vi "SV TDMS Get Function Properties.vi"() -> ()   [LabVIEW 2017]
uses:
  <vilib>/addons/_NISVFA/_Shared subVIs/Controls/NI Channel Properties.ctl
panel:
  in  "file path":path
  out "Array":string[][](array[string])
  out "tdms file":refnum<k34>
  in  "error in (no error)":errorcluster
  out "error out":errorcluster
  out "tdms file out":refnum<k34>
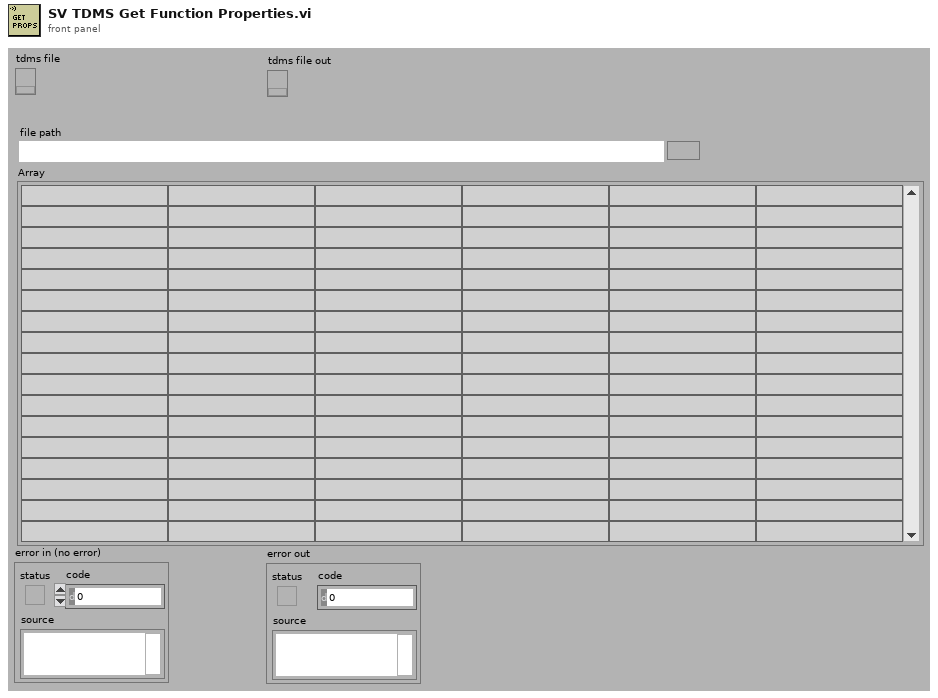
[diagram p1: front panel]
types:
  T1 = typedef "NI Channel Properties.ctl" = u16
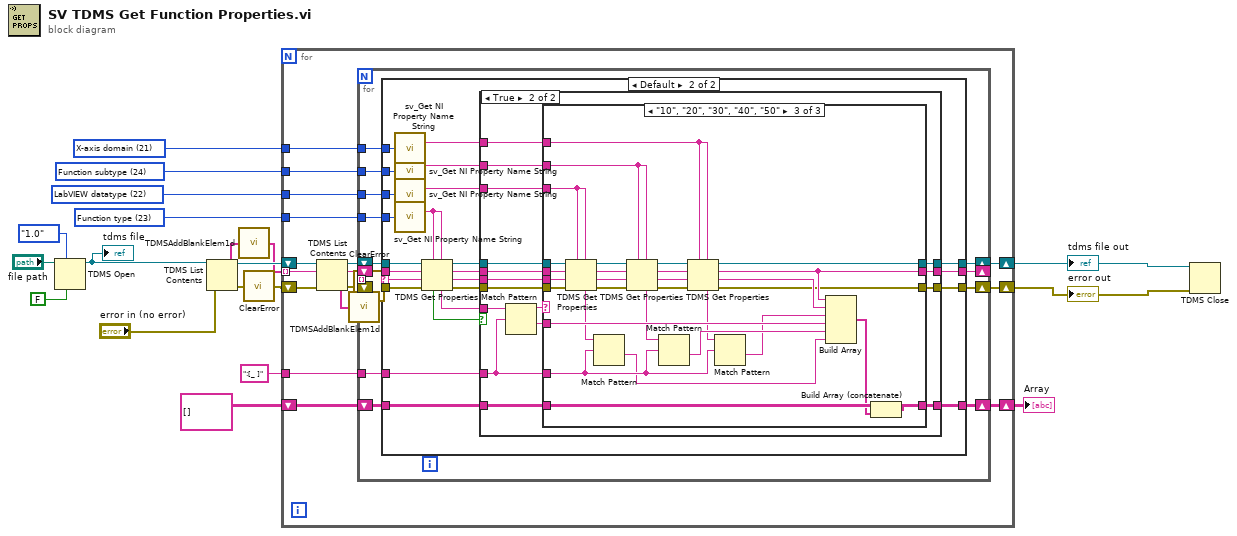
[diagram p0: block diagram]
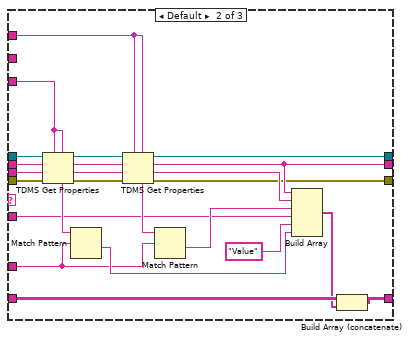
[diagram p5: hidden frame]
diagram:
  w5 = T1 24 items=["Channel name", "Channel description", "Y-axis label", "Y-axis unit string", "X-axis label", "X-axis unit string", "x0", "dx", "Number of samples", "X channel", "Filter settled", "dB reference", "Window", "Window parameter", "Window size", "FFT size", "Peak units", "Spectrum type", "Magnitude scale", "Spectral density", "Sensor sensitivity (mV/EU)", "X-axis domain", "LabVIEW datatype", "Function type", "Function subtype"] ("property")
  w6 = T1 21 items=["Channel name", "Channel description", "Y-axis label", "Y-axis unit string", "X-axis label", "X-axis unit string", "x0", "dx", "Number of samples", "X channel", "Filter settled", "dB reference", "Window", "Window parameter", "Window size", "FFT size", "Peak units", "Spectrum type", "Magnitude scale", "Spectral density", "Sensor sensitivity (mV/EU)", "X-axis domain", "LabVIEW datatype", "Function type", "Component", "Level detector"] ("NI property")
  w7 = T1 22 items=["Channel name", "Channel description", "Y-axis label", "Y-axis unit string", "X-axis label", "X-axis unit string", "x0", "dx", "Number of samples", "X channel", "Filter settled", "dB reference", "Window", "Window parameter", "Window size", "FFT size", "Peak units", "Spectrum type", "Magnitude scale", "Spectral density", "Sensor sensitivity (mV/EU)", "X-axis domain", "LabVIEW datatype", "Function type", "Component", "Level detector"] ("NI property")
  w9 = T1 23 items=["Channel name", "Channel description", "Y-axis label", "Y-axis unit string", "X-axis label", "X-axis unit string", "x0", "dx", "Number of samples", "X channel", "Filter settled", "dB reference", "Window", "Window parameter", "Window size", "FFT size", "Peak units", "Spectrum type", "Magnitude scale", "Spectral density", "Sensor sensitivity (mV/EU)", "X-axis domain", "LabVIEW datatype", "Function type", "Component", "Level detector"] ("NI property")
  n1 = TDMS Open(6:FALSE ("disable buffering? (T)"), 7:enum16{"1.0", "2.0"}."1.0" ("file format version (2.0)"), 11:"file path") -> (3:w10:refnum<k34>)  [unwired: 4 in, 1 out]
  "tdms file" <- w10
  n2 = TDMS List Contents(4:"error in (no error)", 7:w10) -> (0:w1:errorcluster, 2:w2:string[], 3:w19:refnum<k34>)  [unwired: 1 in, 1 out]
  n3 = call <vilib>:"TDMSAddBlankElem1d.vi"("input string array"=w2) -> ("output string array with blank element at the beginning"=w18:string[])
  n4 = call <vilib>:"ClearError.vi"("error in (no error)"=w1) -> ("error out"=w17:errorcluster)
  n5 = for {
    tunnel: w18 -> [w36] mode=indexing
    shift-right: [w33] -> w13
    shift-left: w19 -> [w37]
    shift-right: [w29] -> w14
    shift-left: string[][] [] -> [w30]
    shift-right: [w27] -> w12
    shift-left: w17 -> [w35]
    tunnel: w9 -> [w26]
    tunnel: ":[_ ]" -> [w25]
    tunnel: w7 -> [w24]
    tunnel: w6 -> [w23]
    tunnel: w5 -> [w22]
    n6 = TDMS List Contents(4:w35, 6:w36, 7:w37) -> (0:w20:errorcluster, 1:w21:string[], 2:w31:string, 3:w34:refnum<k34>)
    n7 = call <vilib>:"TDMSAddBlankElem1d.vi"("input string array"=w21) -> ("output string array with blank element at the beginning"=w32:string[])
    n8 = call <vilib>:"ClearError.vi"("error in (no error)"=w20) -> ("error out"=w28:errorcluster)
    n9 = for {
      tunnel: w32 -> [w43] mode=indexing
      shift-right: [w50] -> w33
      shift-left: w34 -> [w51]
      shift-right: [w48] -> _
      shift-left: w31 -> [w49]
      shift-right: [w46] -> w29
      shift-left: w30 -> [w47]
      shift-right: [w44] -> w27
      shift-left: w28 -> [w45]
      tunnel: w26 -> [w42]
      tunnel: w25 -> [w41]
      tunnel: w24 -> [w40]
      tunnel: w23 -> [w39]
      tunnel: w22 -> [w38]
      n10 = case shown="Default" w43 {
        selector: w43 -> [_ w74]
        tunnel: w51 -> [w54 w79]
        tunnel: [w54 w67] -> w50
        tunnel: w49 -> [w55 w78]
        tunnel: [w55 w69] -> w48
        tunnel: w47 -> [w53 w77]
        tunnel: [w53 w76] -> w46
        tunnel: w45 -> [w52 w75]
        tunnel: [w52 w68] -> w44
        tunnel: w42 -> [_ w62]
        tunnel: w41 -> [_ w63]
        tunnel: w40 -> [_ w61]
        tunnel: w39 -> [_ w59]
        tunnel: w38 -> [_ w57]
        frame "" {
        }
        frame Default {
          n11 = call <vilib>:"sv_Get NI Property Name String.vi"("property"=w59) -> ("TDMS property name"=w58:string)  [unwired: 13 in, 1 out]
          n12 = call <vilib>:"sv_Get NI Property Name String.vi"("property"=w57) -> ("TDMS property name"=w56:string)  [unwired: 13 in, 1 out]
          n13 = call <vilib>:"sv_Get NI Property Name String.vi"("property"=w61) -> ("TDMS property name"=w60:string)  [unwired: 13 in, 1 out]
          n14 = call <vilib>:"sv_Get NI Property Name String.vi"("property"=w62) -> ("TDMS property name"=w66:string)  [unwired: 13 in, 1 out]
          n15 = TDMS Get Properties(5:w66, 7:w66, 8:w75, 9:w74, 10:w78, 11:w79) -> (0:w73:errorcluster, 1:w72:string, 2:w71:string, 3:w70:refnum<k34>, 4:w64:string, 6:w65:bool)
          n16 = case shown="True" w65 {
            tunnel: w77 -> [w83 w99]
            tunnel: [w83 w98] -> w76
            tunnel: w73 -> [w82 w97]
            tunnel: w72 -> [_ w96]
            tunnel: w71 -> [w81 w95]
            tunnel: w70 -> [w80 w94]
            tunnel: [w81 w93] -> w69
            tunnel: [w82 w92] -> w68
            tunnel: [w80 w91] -> w67
            tunnel: w64 -> [_ w87]
            tunnel: w63 -> [_ w86]
            tunnel: w60 -> [_ w89]
            tunnel: w58 -> [_ w88]
            tunnel: w56 -> [_ w84]
            frame False {
            }
            frame True {
              n17 = Match Pattern(string=w87, regular expression=w86) -> (before substring=w90:string, after substring=w85:string)  [unwired: 1 in, 2 out]
              n18 = case shown="\"10\", \"20\", \"30\", \"40\", \"50\"" w90 {
                tunnel: w99 -> [w100 w127 w157]
                tunnel: [w100 w126 w156] -> w98
                tunnel: w97 -> [w101 w117 w155]
                tunnel: w96 -> [_ w118 w154]
                tunnel: w95 -> [w102 w119 w153]
                tunnel: w94 -> [w103 w120 w152]
                tunnel: [w102 w123 w151] -> w93
                tunnel: [w101 w121 w149] -> w92
                tunnel: [w103 w124 w148] -> w91
                tunnel: w89 -> [_ w116 w145]
                tunnel: w88 -> [_ w111 w146]
                tunnel: w86 -> [_ w104 w135]
                tunnel: w85 -> [_ w106 w136]
                tunnel: w84 -> [_ _ w128]
                frame "" {
                }
                frame Default {
                  n19 = TDMS Get Properties(5:w116, 7:w116, 8:w117, 9:w118, 10:w119, 11:w120) -> (0:w112:errorcluster, 1:w113:string, 2:w114:string, 3:w115:refnum<k34>, 4:w110:string)  [unwired: 1 out]
                  n20 = Match Pattern(string=w110, regular expression=w104) -> (after substring=w105:string)  [unwired: 1 in, 3 out]
                  n21 = TDMS Get Properties(5:w111, 7:w111, 8:w112, 9:w113, 10:w114, 11:w115) -> (0:w121:errorcluster, 1:w122:string, 2:w123:string, 3:w124:refnum<k34>, 4:w108:string)  [unwired: 1 out]
                  n22 = Match Pattern(string=w108, regular expression=w104) -> (after substring=w107:string)  [unwired: 1 in, 3 out]
                  n23 = Build Array(w123, w122, w107, w106, "Value" ("element"), w105) -> (w125:string[])
                  n24 = Build Array (concatenate)(w127, w125) -> (w126:string[][])
                }
                frame "10", "20", "30", "40", "50" {
                  n25 = TDMS Get Properties(5:w145, 7:w145, 8:w155, 9:w154, 10:w153, 11:w152) -> (0:w144:errorcluster, 1:w143:string, 2:w142:string, 3:w141:refnum<k34>, 4:w134:string)  [unwired: 1 out]
                  n26 = Match Pattern(string=w134, regular expression=w135) -> (after substring=w133:string)  [unwired: 1 in, 3 out]
                  n27 = TDMS Get Properties(5:w128, 7:w128, 8:w144, 9:w143, 10:w142, 11:w141) -> (0:w137:errorcluster, 1:w138:string, 2:w139:string, 3:w140:refnum<k34>, 4:w132:string)  [unwired: 1 out]
                  n28 = Match Pattern(string=w132, regular expression=w135) -> (after substring=w131:string)  [unwired: 1 in, 3 out]
                  n29 = TDMS Get Properties(5:w146, 7:w146, 8:w137, 9:w138, 10:w139, 11:w140) -> (0:w149:errorcluster, 1:w150:string, 2:w151:string, 3:w148:refnum<k34>, 4:w130:string)  [unwired: 1 out]
                  n30 = Match Pattern(string=w130, regular expression=w135) -> (after substring=w129:string)  [unwired: 1 in, 3 out]
                  n31 = Build Array(w151, w150, w129, w136, w131, w133) -> (w147:string[])
                  n32 = Build Array (concatenate)(w157, w147) -> (w156:string[][])
                }
              }
            }
          }
        }
      }
    }
  }
  "tdms file out" <- w13
  "error out" <- w12
  "Array" <- w14
  n33 = TDMS Close(8:w12, 11:w13) -> ()  [unwired: 2 out]
